vi "Ramp_Field.vi"(5 "Set Field (T) in":dbl, 6 "Sweep Rate (T/min)":dbl, 7 "V/I (Ohm)":dbl, 8 "error in (no error)":errorcluster, 9 "Magnet":bool, 10 "B/V (T/V)":dbl, 11 "VISA Refnum in":refnum<visa-resource-name>) -> (0 "error out":errorcluster, 2 "Actual Voltage (V)":dbl, 3 "Set Field (T) out":dbl)   [LabVIEW 2015]
uses:
  <vilib>/express/express arith-compare/Formula/XNode/ExpressFormulaBlockNode.xnode
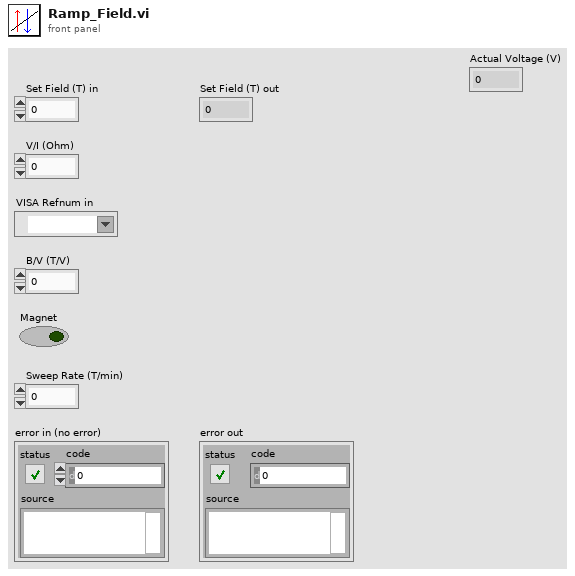
[diagram p1: front panel]
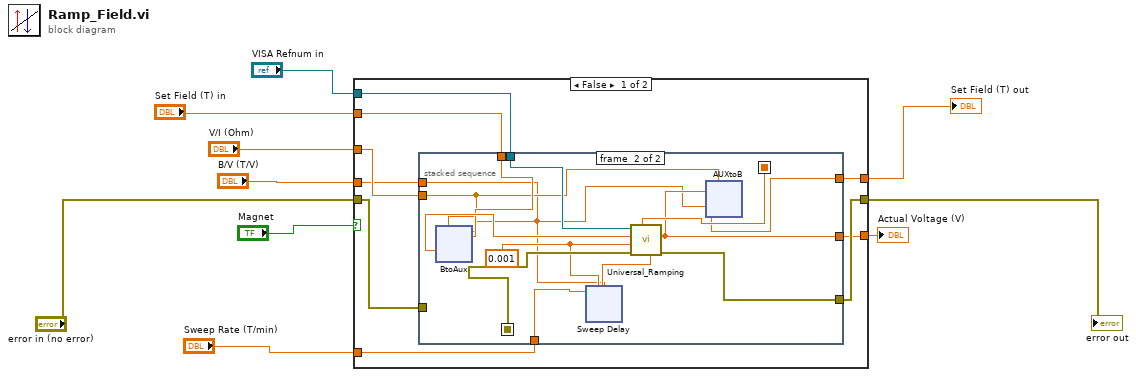
[diagram p0: block diagram]
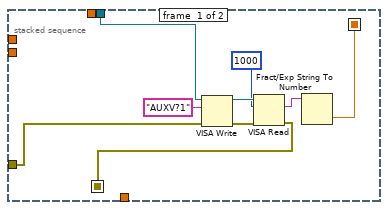
[diagram p2: hidden frame]
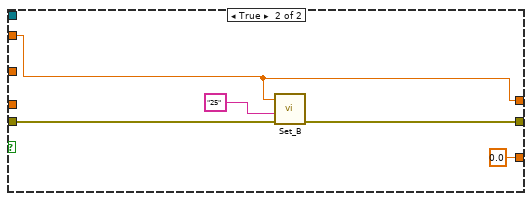
[diagram p3: hidden frame]
diagram:
  n1 = case shown="False" "Magnet" {
    tunnel: [w18 w82] -> w2
    tunnel: "error in (no error)" -> [w19 w81]
    tunnel: "Set Field (T) in" -> [w17 w79]
    tunnel: "V/I (Ohm)" -> [w16 _]
    tunnel: "B/V (T/V)" -> [w15 _]
    tunnel: "Sweep Rate (T/min)" -> [w14 _]
    tunnel: [w13 w79] -> w8
    tunnel: "VISA Refnum in" -> [w12 _]
    tunnel: [w11 0.0 ("Actual Voltage (V)")] -> w1
    frame False {
      n2 = stacked-sequence {
        seq-local: [w22 _] -> [_ w39]
        seq-local: [w20 _] -> [_ w37]
        tunnel: w19 -> [w24 _]
        tunnel: [_ w40] -> w18
        tunnel: w12 -> [w21 w38]
        tunnel: w17 -> [_ w35]
        tunnel: w16 -> [_ w34]
        tunnel: w15 -> [_ w29]
        tunnel: w14 -> [_ w33]
        tunnel: [_ w32] -> w13
        tunnel: [_ w31] -> w11
        frame #0 {
          n3 = VISA Write(VISA resource name=w21, write buffer="AUXV?1", error in (no error)=w24) -> (VISA resource name out=w28:refnum<visa-resource-name>, error out=w23:errorcluster)  [unwired: 1 out]
          n4 = VISA Read(VISA resource name=w28, byte count=u32 1000, error in (no error)=w23) -> (read buffer=w25:string, error out=w22:errorcluster)  [unwired: 2 out]
          n5 = Fract/Exp String To Number(string=w25) -> (number=w20:dbl)  [unwired: 3 in, 1 out]
        }
        frame #1 {
          w30 = 0.001 ("Voltage Step (V)")
          n6 = xnode "BtoAux"("BpV"=w29, "Rm"=w34, "B"=w35) -> ("Result"=w36:dbl)  [unwired: 1 in, 1 out]
          n7 = xnode "Sweep Delay"("SweepRate"=w33, "Resolution"=w30, "BpV"=w29) -> ("Result"=w41:dbl)  [unwired: 1 in, 1 out]
          n8 = call "Universal_Ramping.vi"("milliseconds to wait"=w41, "Initial Voltage (V)"=w37, "error in (no error)"=w39, "Voltage Step (V)"=w30, "Final Voltage (V)"=w36, "VISA resource name"=w38) -> ("error out"=w40:errorcluster, "Actual Voltage (V)"=w31:dbl)  [unwired: 3 in, 1 out]
          n9 = xnode "AUXtoB"("BpV"=w29, "Rm"=w34, "Aux"=w31) -> ("Result"=w32:dbl)  [unwired: 1 in, 1 out]
        }
      }
    }
    frame True {
      n10 = call "Set_B.vi"("error in (no error)"=w81, "address string"="25", "Set Field (T)"=w79) -> ("error out"=w82:errorcluster)  [unwired: 8 in]
    }
  }
  "Set Field (T) out" <- w8
  "error out" <- w2
  "Actual Voltage (V)" <- w1
